vi "ParseControlsForHelp.vi"(6 "Help Information":T1, 7 "Device Name":string, 8 "error in (no error)":errorcluster, 9 "Property Bundle":cluster{"Name":string, "Value":variant}[](array[cluster]), 10 "Control Refs":refnum<vi>[](array[refnum]), 11 "String in":string) -> (0 "error out":errorcluster, 3 "String out":string)   [LabVIEW 2021]
uses:
  <vilib>/myRIO/Common/Express VI Framework/xctls/myRIO Channel List/myRIO Channel List.xctl
  <vilib>/myRIO/Common/Express VI Framework/xctls/myRIO Channel Name/myRIO Channel Name.xctl
panel:
  out "Value":variant
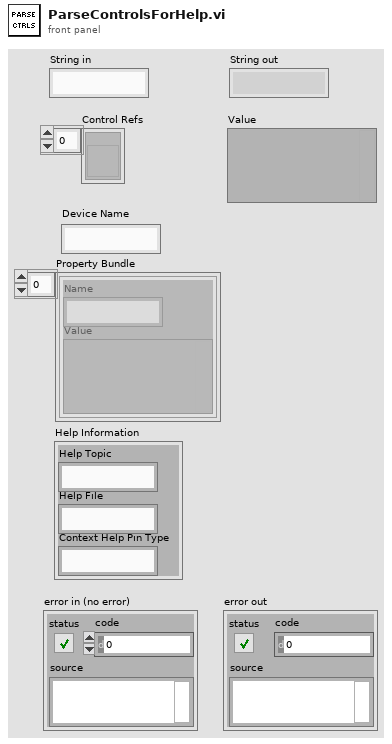
[diagram p1: front panel]
types:
  T1 = cluster{"Help Topic":string, "Help File":string, "Context Help Pin Type":string}
  T2 = enum8{"Enabled", "Disabled", "Disabled and Grayed Out"}
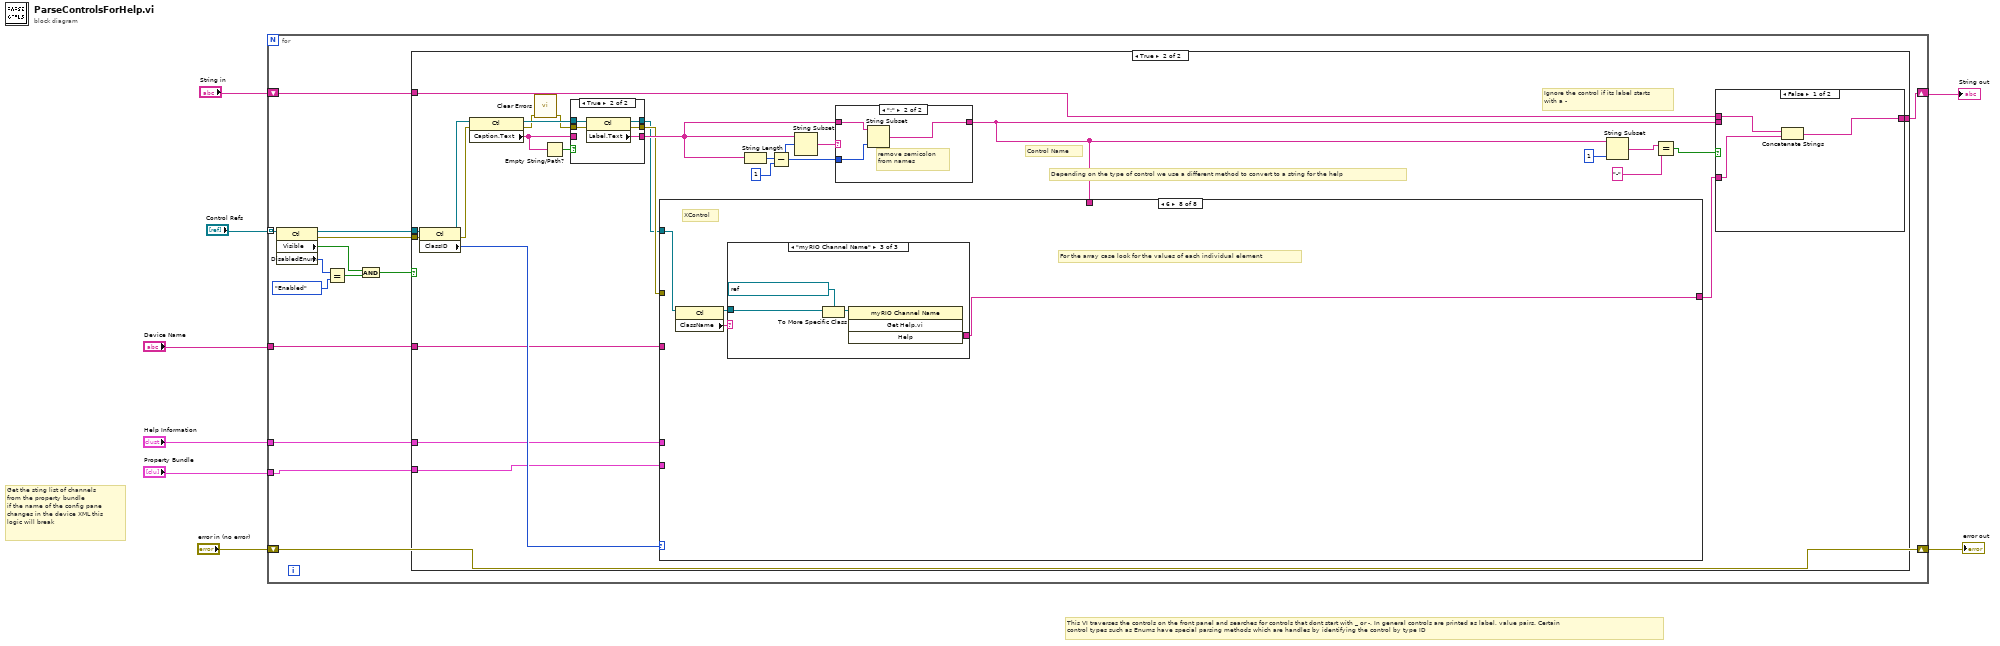
[diagram p0: block diagram]
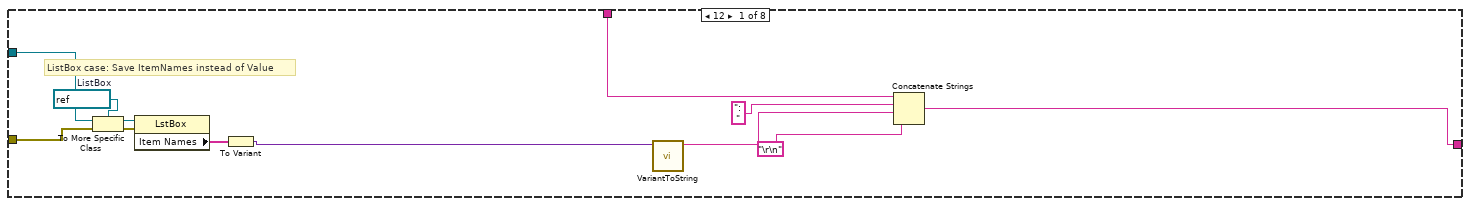
[diagram p6: hidden frame]
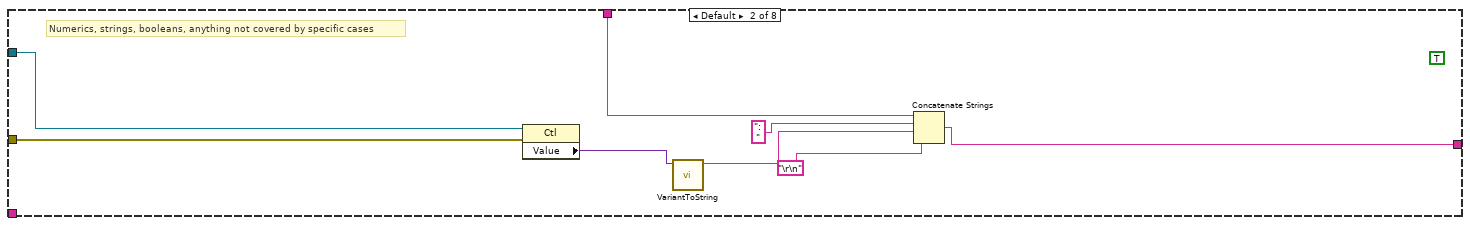
[diagram p7: hidden frame]
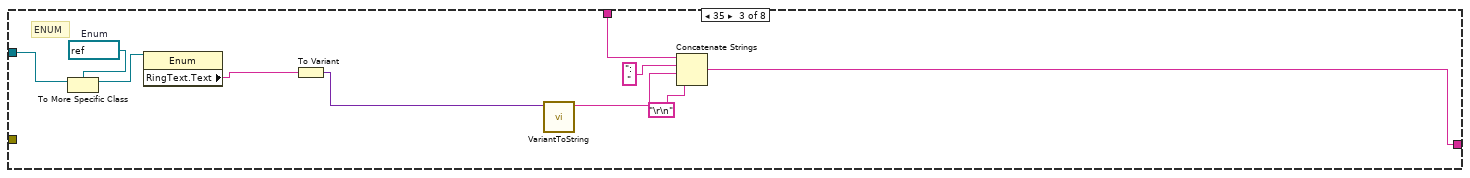
[diagram p8: hidden frame]
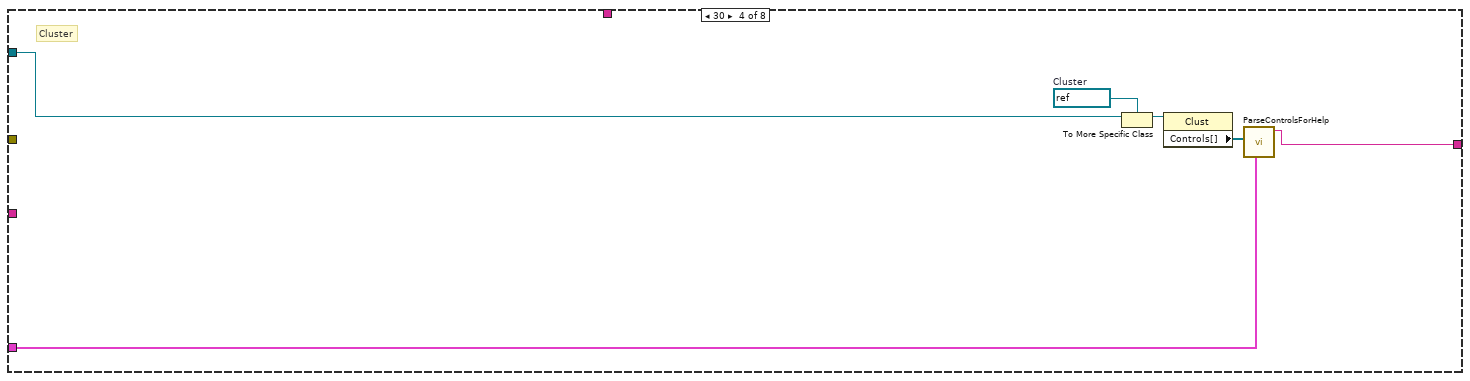
[diagram p9: hidden frame]
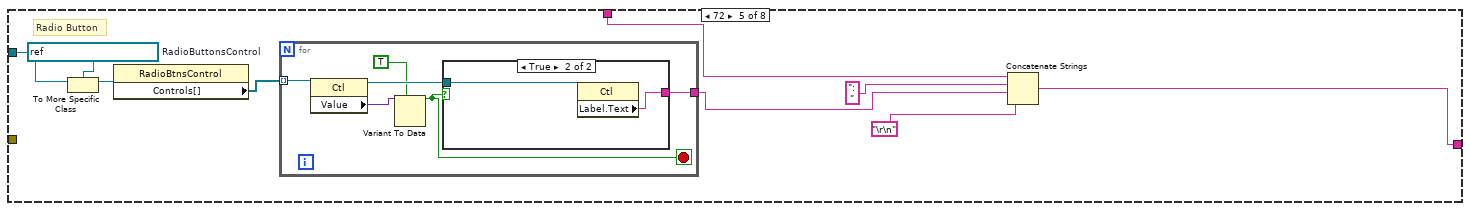
[diagram p10: hidden frame]
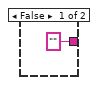
[diagram p11: hidden frame]
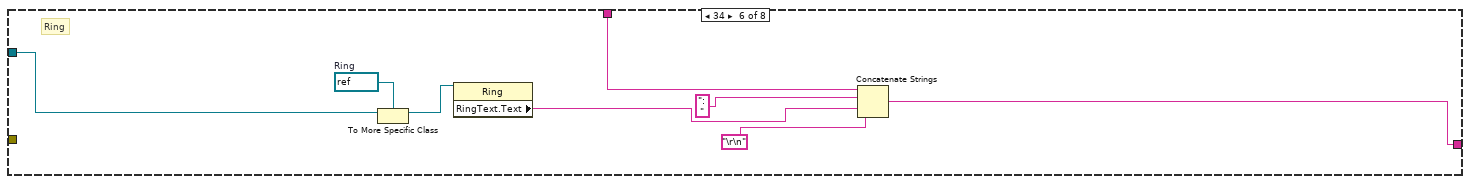
[diagram p12: hidden frame]
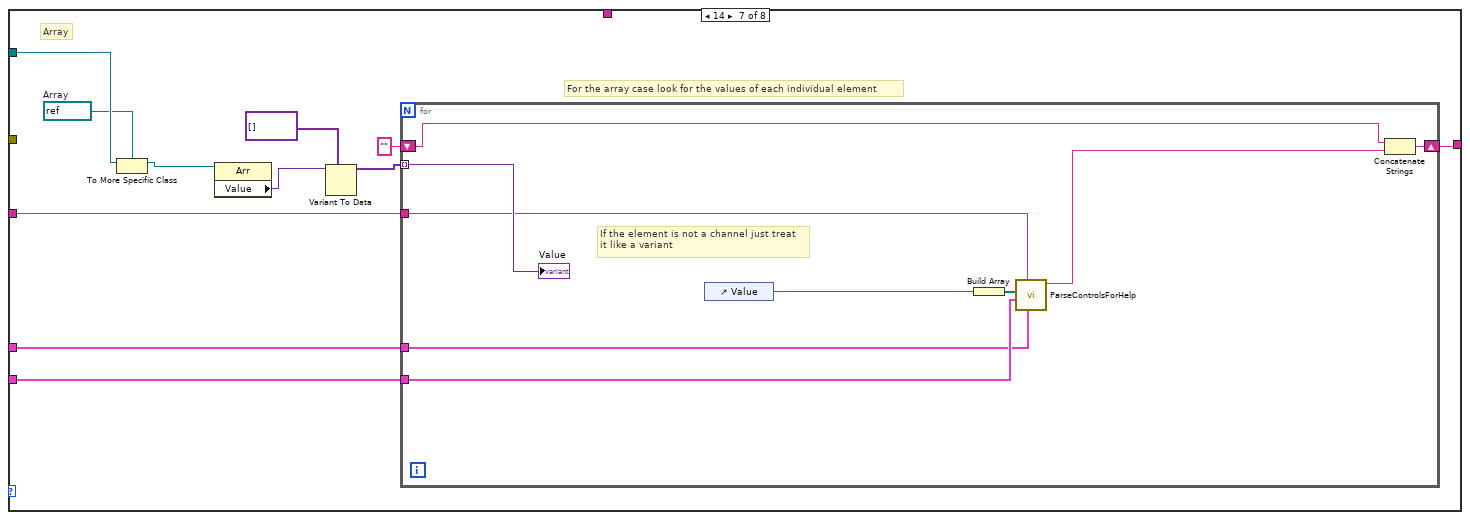
[diagram p13: hidden frame]
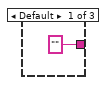
[diagram p14: hidden frame]
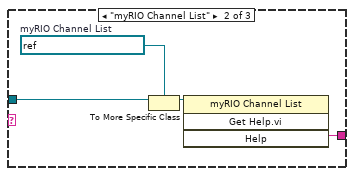
[diagram p15: hidden frame]
diagram:
  # "Get the sting list of channels\nfrom the property bundle\nif the name of the config pane\nchanges in the device XML this\nlogic will break"
  # "This VI traverses the controls on the front panel and searches for controls that dont start with _ or -. In general controls are printed as label, value pairs. Certain\ncontrol types such as Enums have special parsing methods which are handles by identifying the control by type ID"
  n1 = for {
    tunnel: "Control Refs" -> [w15] mode=indexing
    shift-right: [w22] -> w4
    shift-left: "error in (no error)" -> [w22]
    shift-right: [w20] -> w8
    shift-left: "String in" -> [w21]
    tunnel: "Device Name" -> [w19]
    tunnel: "Property Bundle" -> [w18]
    tunnel: "Help Information" -> [w14]
    n2 = property class="Ctl"(reference=w15) -> (reference out=w16:refnum<vi>, error out=w17:errorcluster, "Visible"=w10:bool, "DisabledEnum"=w13:T2)  [unwired: 1 in]
    n3 = Equal?(x=w13, y=T2."Enabled" ("Disabled")) -> (x = y?=w11:bool)
    n4 = And(x=w10, y=w11) -> (x .and. y?=w9:bool)
    n5 = case shown="True" w9 {
      tunnel: w21 -> [w23 w50]
      tunnel: [w23 w41] -> w20
      tunnel: w19 -> [_ w39]
      tunnel: w18 -> [_ w38]
      tunnel: w17 -> [_ w36]
      tunnel: w16 -> [_ w35]
      tunnel: w14 -> [_ w34]
      frame False {
        # "Control is disabled.\nDon't display context help for disabled controls"
      }
      frame True {
        # "Depending on the type of control we use a different method to convert to a string for the help"
        # "Control Name"
        # "Ignore the control if its label starts\nwith a -"
        n6 = property class="Ctl"(reference=w35, error in=w36) -> (reference out=w30:refnum<vi>, error out=w33:errorcluster, "ClassID"=w51:u32)
        n7 = property class="Ctl"(reference=w30, error in=w33) -> (reference out=w32:refnum<vi>, error out=w27:errorcluster, "Caption.Text"=w29:string)
        n8 = call <vilib>:"Clear Errors.vi"("error in (no error)"=w27) -> ("error out"=w26:errorcluster)  [unwired: 5 in, 1 out]
        n9 = Empty String/Path?(string/path=w29) -> (empty?=w28:bool)
        n10 = case shown="True" w28 {
          tunnel: w32 -> [w52 w59]
          tunnel: [w54 w58] -> w31
          tunnel: w29 -> [w54 _]
          tunnel: w26 -> [w53 w57]
          tunnel: [w53 w56] -> w25
          tunnel: [w52 w55] -> w24
          frame False {
          }
          frame True {
            n11 = property class="Ctl"(reference=w59, error in=w57) -> (reference out=w55:refnum<vi>, error out=w56:errorcluster, "Label.Text"=w58:string)
          }
        }
        n12 = String Length(string=w31) -> (length=w45:i32)
        n13 = Subtract(x=w45, y=1) -> (x-y=w42:i32)
        n14 = String Subset(string=w31, offset (0)=w42) -> (substring=w43:string)  [unwired: 1 in]
        n15 = case shown="\":\"" w43 {
          tunnel: w31 -> [w60 w63]
          tunnel: [w60 w61] -> w37
          tunnel: w42 -> [_ w62]
          frame Default {
          }
          frame ":" {
            # "remove semicolon\nfrom names"
            n16 = String Subset(string=w63, length (rest)=w62) -> (substring=w61:string)  [unwired: 1 in]
          }
        }
        n17 = case shown="6" w51 {
          tunnel: w24 -> [w79 w87 w96 w101 w111 w128 w140 w153]
          tunnel: w25 -> [w74 w86 _ _ _ _ _ _]
          tunnel: [w68 w81 w88 w99 w104 w122 w136 w151] -> w40
          tunnel: w39 -> [_ _ _ _ _ _ w133 _]
          tunnel: w38 -> [_ _ _ _ _ _ w132 _]
          tunnel: w37 -> [w70 w80 w90 _ w106 w124 _ _]
          tunnel: w34 -> [_ _ _ w98 _ _ w131 _]
          frame 12 {
            w78 = refnum<vi> refnum  # ListBox
            # "ListBox case: Save ItemNames instead of Value"
            n18 = To More Specific Class(target class=w78, reference=w79, error in=w74) -> (specific class reference=w77:refnum<vi>, error out=w76:errorcluster)
            n19 = property class="LstBox"(reference=w77, error in=w76) -> ("Item Names"=w75:string[])  [unwired: 2 out]
            n20 = To Variant(anything=w75) -> (Variant=w69:variant)
            n21 = call <vilib>:"VariantToString.vi"("Variant"=w69) -> ("String"=w72:string)  [unwired: 10 in]
            n22 = Concatenate Strings(w70, ": " ("string"), w72, "\r\n") -> (w68:string)
          }
          frame Default {
            (unwired) TRUE ("Use Variant?")
            # "Numerics, strings, booleans, anything not covered by specific cases"
            n23 = property class="Ctl"(reference=w87, error in=w86) -> ("Value"=w82:variant)  [unwired: 2 out]
            n24 = call <vilib>:"VariantToString.vi"("Variant"=w82) -> ("String"=w84:string)  [unwired: 10 in]
            n25 = Concatenate Strings(w80, ": " ("string"), w84, "\r\n") -> (w81:string)
          }
          frame 35 {
            w97 = refnum<vi> refnum  # Enum
            # "ENUM"
            n26 = To More Specific Class(target class=w97, reference=w96) -> (specific class reference=w95:refnum<vi>)  [unwired: 1 in, 1 out]
            n27 = property on="Property Node" class="Enum"(reference=w95) -> ("RingText.Text"=w94:string)  [unwired: 1 in, 2 out]
            n28 = To Variant(anything=w94) -> (Variant=w89:variant)
            n29 = call <vilib>:"VariantToString.vi"("Variant"=w89) -> ("String"=w92:string)  [unwired: 10 in]
            n30 = Concatenate Strings(w90, ": " ("string"), w92, "\r\n") -> (w88:string)
          }
          frame 30 {
            w103 = refnum<vi> refnum  # Cluster
            # "Cluster"
            n31 = To More Specific Class(target class=w103, reference=w101) -> (specific class reference=w102:refnum<vi>)  [unwired: 1 in, 1 out]
            n32 = property class="Clust"(reference=w102) -> ("Controls[]"=w100:refnum<vi>[])  [unwired: 1 in, 2 out]
            n33 = call <vilib>:"ParseControlsForHelp.vi"("Help Information"=w98, "Control Refs"=w100) -> ("String out"=w99:string)  [unwired: 8 in, 1 out]
          }
          frame 72 {
            w112 = refnum<vi> refnum  # RadioButtonsControl
            # "Radio Button"
            n34 = To More Specific Class(target class=w112, reference=w111) -> (specific class reference=w110:refnum<vi>)  [unwired: 1 in, 1 out]
            n35 = property on="Property Node" class="RadioBtnsControl"(reference=w110) -> ("Controls[]"=w109:refnum<vi>[])  [unwired: 1 in, 2 out]
            n36 = for {
              tunnel: w109 -> [w118] mode=indexing
              tunnel: [w114] -> w105
              stop <- w113 stop-if-true
              n37 = property class="Ctl"(reference=w118) -> (reference out=w117:refnum<vi>, "Value"=w116:variant)  [unwired: 1 in, 1 out]
              n38 = Variant To Data(type=TRUE, Variant=w116) -> (data=w113:bool)  [unwired: 1 in, 1 out]
              n39 = case shown="True" w113 {
                tunnel: w117 -> [_ w121]
                tunnel: ["" ("Label.Text") w120] -> w114
                frame False {
                }
                frame True {
                  n40 = property class="Ctl"(reference=w121) -> ("Label.Text"=w120:string)  [unwired: 1 in, 2 out]
                }
              }
            }
            n41 = Concatenate Strings(w106, ": " ("string"), w105, "\r\n") -> (w104:string)
          }
          frame 34 {
            w129 = refnum<vi> refnum  # Ring
            # "Ring"
            n42 = To More Specific Class(target class=w129, reference=w128) -> (specific class reference=w127:refnum<vi>)  [unwired: 1 in, 1 out]
            n43 = property on="Property Node" class="Ring"(reference=w127) -> ("RingText.Text"=w123:string)  [unwired: 1 in, 2 out]
            n44 = Concatenate Strings(w124, ": " ("string"), w123, "\r\n") -> (w122:string)
          }
          frame 14 {
            w134 = refnum<vi> refnum  # Array
            # "For the array case look for the values of each individual element"
            # "Array"
            n45 = To More Specific Class(target class=w134, reference=w140) -> (specific class reference=w139:refnum<vi>)  [unwired: 1 in, 1 out]
            n46 = property class="Arr"(reference=w139) -> ("Value"=w135:variant)  [unwired: 1 in, 2 out]
            n47 = Variant To Data(type=variant[] [], Variant=w135) -> (data=w137:variant[])  [unwired: 1 in, 1 out]
            n48 = for {
              tunnel: w137 -> [w146] mode=indexing
              shift-right: [w149] -> w136
              shift-left: "" -> [w148]
              tunnel: w133 -> [w145]
              tunnel: w132 -> [w144]
              tunnel: w131 -> [w143]
              # "If the element is not a channel just treat\nit like a variant"
              n49 = control-ref of="Value"() -> (w142:refnum<vi>)
              n50 = Build Array(w142) -> (w141:refnum<vi>[])
              n51 = call <vilib>:"ParseControlsForHelp.vi"("Help Information"=w143, "Device Name"=w145, "Property Bundle"=w144, "Control Refs"=w141) -> ("String out"=w147:string)  [unwired: 6 in, 1 out]
              n52 = Concatenate Strings(w148, w147) -> (w149:string)
              "Value" <- w146
            }
          }
          frame 6 {
            # "For the array case look for the values of each individual element"
            # "XControl"
            n53 = property class="Ctl"(reference=w153) -> (reference out=w152:refnum<vi>, "ClassName"=w150:string)  [unwired: 1 in, 1 out]
            n54 = case shown="\"myRIO Channel Name\"" w150 {
              tunnel: w152 -> [_ w157 w162]
              tunnel: ["" ("Help") w155 w159] -> w151
              frame Default {
              }
              frame "myRIO Channel List" {
                w158 = refnum<vi> refnum  # myRIO Channel List
                n55 = To More Specific Class(target class=w158, reference=w157) -> (specific class reference=w156:refnum<vi>)  [unwired: 1 in, 1 out]
                n56 = invoke class="myRIO Channel List" method="Get Help.vi"(reference=w156) -> ("Help"=w155:string)  [unwired: 3 in, 3 out]
              }
              frame "myRIO Channel Name" {
                n57 = To More Specific Class(target class=refnum<vi> refnum ("myRIO Channel Name"), reference=w162) -> (specific class reference=w161:refnum<vi>)  [unwired: 1 in, 1 out]
                n58 = invoke class="myRIO Channel Name" method="Get Help.vi"(reference=w161) -> ("Help"=w159:string)  [unwired: 3 in, 3 out]
              }
            }
          }
        }
        n59 = String Subset(string=w37, length (rest)=1 ("length (rest)")) -> (substring=w48:string)  [unwired: 1 in]
        n60 = Equal?(x=w48, y="-") -> (x = y?=w46:bool)
        n61 = case shown="False" w46 {
          tunnel: w50 -> [w66 w67]
          tunnel: [w65 w67] -> w41
          tunnel: w37 -> [_ _]
          tunnel: w40 -> [w64 _]
          frame False {
            n62 = Concatenate Strings(w66, w64) -> (w65:string)
          }
          frame True {
            # "Exclude controls\nwhose label starts with\n- from help"
          }
        }
      }
    }
  }
  "String out" <- w8
  "error out" <- w4
